vi "resize window.vi"(8 "don't grow front panels":bool, 9 "y (600)":i16=600, 10 "x (800)":i16=800, 11 "vis":refnum<vi>[](array[refnum])) -> (0 "error report":errorcluster[](array[cluster]))   [LabVIEW 2013, in "cosmetic changes.lvclass"]
uses:
  cosmetic changes.lvclass
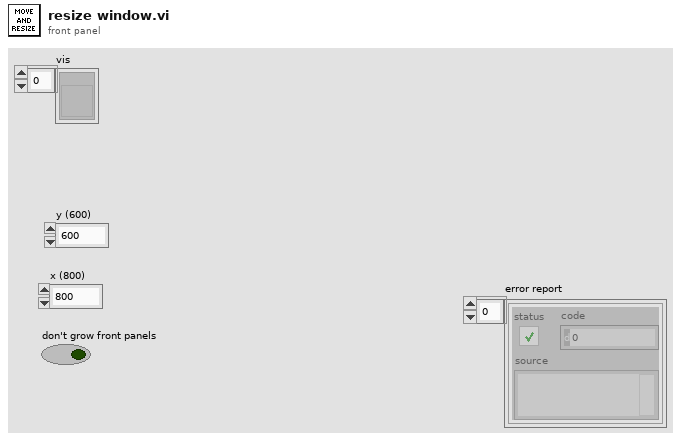
[diagram p1: front panel]
types:
  T1 = typedef "LVRectTypeDef.ctl" = cluster{"Left":i16, "Top":i16, "Right":i16, "Bottom":i16}
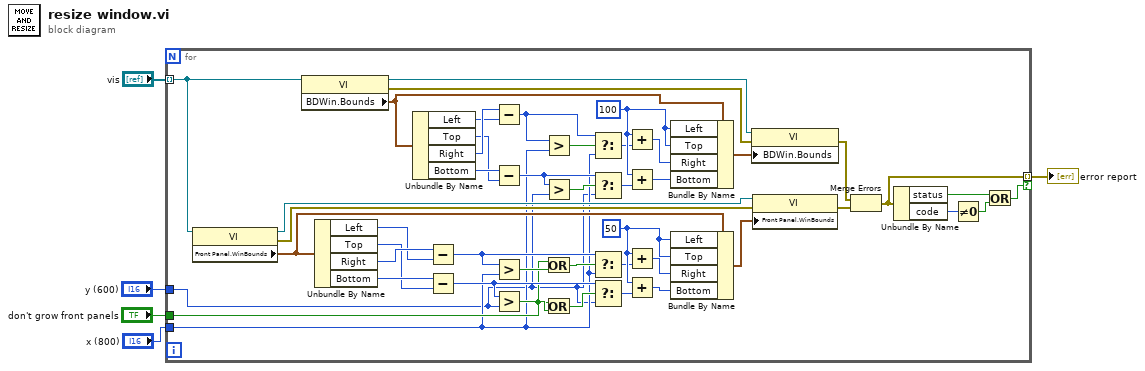
[diagram p0: block diagram]
diagram:
  n1 = for {
    tunnel: "vis" -> [w12] mode=indexing
    tunnel: [w8] -> w4 mode=indexing if=w49
    tunnel: "don't grow front panels" -> [w11]
    tunnel: "y (600)" -> [w6]
    tunnel: "x (800)" -> [w7]
    w29 = i16 50 ("Left")
    w30 = i16 100 ("Left")
    n2 = property class="VI"(reference=w12) -> (reference out=w20:refnum<vi>, error out=w19:errorcluster, "Front Panel.WinBounds"=w15:T1)  [unwired: 1 in]
    n3 = property class="VI"(reference=w12) -> (reference out=w47:refnum<vi>, error out=w48:errorcluster, "BDWin.Bounds"=w18:T1)  [unwired: 1 in]
    n4 = Unbundle By Name(w15) -> ("Left"=w35:i16, "Top"=w31:i16, "Right"=w36:i16, "Bottom"=w32:i16)
    n5 = Unbundle By Name(w18) -> ("Left"=w45:i16, "Top"=w33:i16, "Right"=w46:i16, "Bottom"=w34:i16)
    n6 = Subtract(x=w36, y=w35) -> (x-y=w38:i16)
    n7 = Subtract(x=w32, y=w31) -> (x-y=w39:i16)
    n8 = Subtract(x=w46, y=w45) -> (x-y=w43:i16)
    n9 = Subtract(x=w34, y=w33) -> (x-y=w42:i16)
    n10 = Greater?(x=w38, y=w7) -> (0:w37:bool)
    n11 = Greater?(x=w39, y=w6) -> (0:w40:bool)
    n12 = Greater?(x=w43, y=w7) -> (0:w44:bool)
    n13 = Greater?(x=w42, y=w6) -> (0:w41:bool)
    n14 = Or(x=w11, y=w37) -> (x .or. y?=w14:bool)
    n15 = Or(x=w11, y=w40) -> (x .or. y?=w13:bool)
    n16 = Select(t=w43, s=w44, f=w7) -> (s? t:f=w25:i16)
    n17 = Select(t=w42, s=w41, f=w6) -> (s? t:f=w26:i16)
    n18 = Select(t=w38, s=w14, f=w7) -> (s? t:f=w28:i16)
    n19 = Select(t=w39, s=w13, f=w6) -> (s? t:f=w27:i16)
    n20 = Add(x=w30, y=w25) -> (x+y=w24:i16)
    n21 = Add(x=w30, y=w26) -> (x+y=w23:i16)
    n22 = Add(x=w29, y=w28) -> (x+y=w22:i16)
    n23 = Add(x=w29, y=w27) -> (x+y=w21:i16)
    n24 = Bundle By Name(cluster=w18, "Left"=w30, "Top"=w30, "Right"=w24, "Bottom"=w23) -> (w17:T1)
    n25 = Bundle By Name(cluster=w15, "Left"=w29, "Top"=w29, "Right"=w22, "Bottom"=w21) -> (w16:T1)
    n26 = property class="VI"(reference=w47, error in=w48, "BDWin.Bounds"=w17) -> (error out=w10:errorcluster)  [unwired: 1 out]
    n27 = property class="VI"(reference=w20, error in=w19, "Front Panel.WinBounds"=w16) -> (error out=w9:errorcluster)  [unwired: 1 out]
    n28 = Merge Errors(w10, w9) -> (w8:errorcluster)
    n29 = Unbundle By Name(w8) -> ("status"=w52:bool, "code"=w51:i32)
    n30 = Not Equal To 0?(x=w51) -> (x != 0?=w50:bool)
    n31 = Or(x=w52, y=w50) -> (x .or. y?=w49:bool)
  }
  "error report" <- w4
